vi "MFC Check Valve Mode.vi"(11 "Valve Mode":string(combo)) -> (3 "Valve Mode out":string)   [LabVIEW 2020, in "MRC Module.lvlib"]
uses:
  MRC Module.lvlib
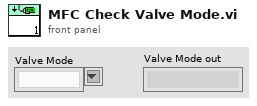
[diagram p1: front panel]
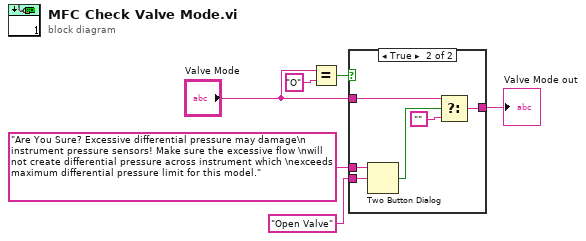
[diagram p0: block diagram]
diagram:
  n1 = Equal?(x="Valve Mode", y="O") -> (x = y?=w1:bool)
  n2 = case shown="True" w1 {
    tunnel: "Valve Mode" -> [w7 w13]
    tunnel: [w7 w11] -> w6
    tunnel: "Are You Sure? Excessive differential pressure may damage\n instrument pressure sensors! Make sure the excessive flow \nwill not create differential pressure across instrument which \nexceeds maximum differential pressure limit for this model." -> [_ w9]
    tunnel: "Open Valve" -> [_ w8]
    frame False {
    }
    frame True {
      n3 = Two Button Dialog(message=w9, 2:w8) -> (T button?=w10:bool)  [unwired: 1 in]
      n4 = Select(t=w13, s=w10, f="") -> (s? t:f=w11:string)
    }
  }
  "Valve Mode out" <- w6
